vi "StringAsArray.vi"(8 "error in":errorcluster, 11 "Array In":string[](array[string])) -> (0 "error out":errorcluster, 3 "ArrayAsValue":string)   [LabVIEW 2009]
uses:
  SetScalarValue/StringAsValue.vi
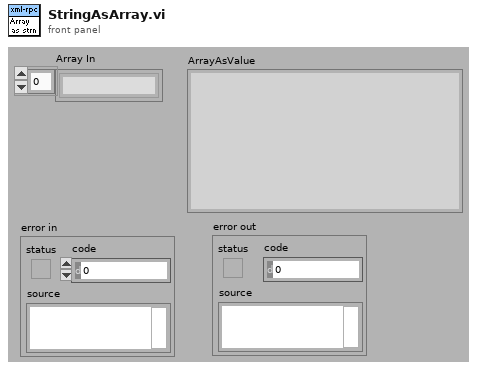
[diagram p1: front panel]
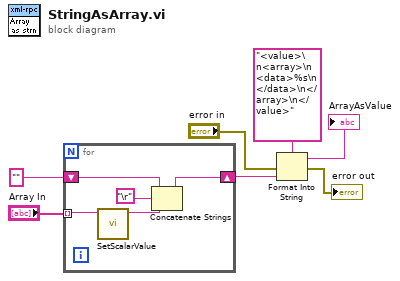
[diagram p0: block diagram]
diagram:
  n1 = for {
    tunnel: "Array In" -> [w12] mode=indexing
    shift-right: [w10] -> w5
    shift-left: "" -> [w11]
    n2 = call-poly "SetScalarValue.vi"("scalar value (string)"=w12) -> ("scalar string"=w8:string)  [unwired: 9 in, 1 out]
    n3 = Concatenate Strings(w11, "\r", w8) -> (w10:string)
  }
  n4 = Format Into String(format string="<value>\n<array>\n  <data>%s\n  </data>\n</array>\n</value>", error in="error in", w5) -> (resulting string=→"ArrayAsValue":string, error out=→"error out":errorcluster)  [unwired: 1 in]
